vi "ConfigSilos.vi"() -> ()   [LabVIEW 2014]
doc: "The LabJack T7 offers several AIN Extended Features. One such feature is called FlexRMS. Data acquired at a specified AIN Channel are buffered, on-board calculations (rms,range,average) are performed and the results are written to AIN-EF registers. This VI configures the Flex RMS EF to avoid using external computational resources whilst seeking averaged data. THE SCAN DURATION CANNOT EXCEED 180 ms!!"
panel:
  in  "Remote Port":u16=502
  in  "Remote IP Address":string="192.168.126.147"
  in  "Num AI Channels":dbl=16.0
  out "Scan Duration (ms)":dbl=180.0
  in  "Scan Rate (Hz)":sgl=6000.0
  in  "Hysteresis":u32=100
  in  "NumScans":u32=1080
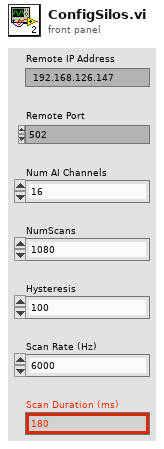
[diagram p1: front panel]
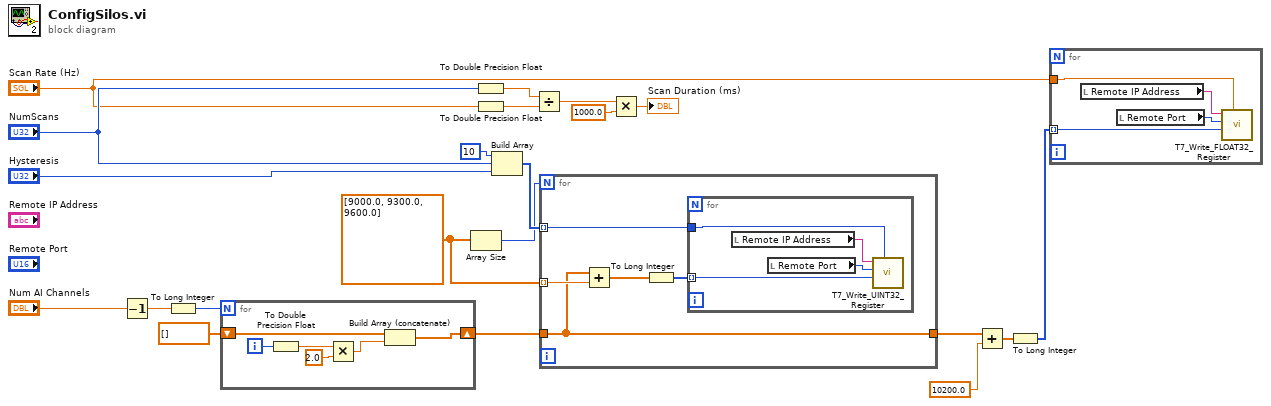
[diagram p0: block diagram]
diagram:
  w13 = dbl[] [9000.0, 9300.0, 9600.0]
  n1 = Decrement(x="Num AI Channels") -> (x-1=w18:dbl)
  n2 = To Long Integer(number=w18) -> (32bit integer=w19:i32)
  n3 = for {
    N: w19 -> [_]
    shift-right: [w26] -> w17
    shift-left: dbl[] [] -> [w25]
    i -> [w27]
    n4 = To Double Precision Float(number=w27) -> (double precision float=w23:dbl)
    n5 = Multiply(x=w23, y=2.0) -> (x*y=w22:dbl)
    n6 = Build Array (concatenate)(w25, w22) -> (w26:dbl[])
  }
  n7 = Array Size(array=w13) -> (size(s)=w12:i32)
  n8 = To Double Precision Float(number="NumScans") -> (double precision float=w3:dbl)
  n9 = To Double Precision Float(number="Scan Rate (Hz)") -> (double precision float=w2:dbl)
  n10 = Build Array(u32 10 ("UINT32 to Write"), "NumScans", "Hysteresis") -> (w14:u32[])
  n11 = Divide(x=w3, y=w2) -> (x/y=w5:dbl)
  n12 = for {
    N: w12 -> [_]
    tunnel: w13 -> [w30] mode=indexing
    tunnel: w17 -> [w28]
    tunnel: w14 -> [w29] mode=indexing
    tunnel: [w28] -> w9
    n13 = Add(x=w28, y=w30) -> (x+y=w31:dbl[])
    n14 = To Long Integer(number=w31) -> (32bit integer=w32:i32[])
    n15 = for {
      tunnel: w32 -> [w35] mode=indexing
      tunnel: w29 -> [w34]
      n16 = local read "Remote IP Address"() -> (w36:string)
      n17 = local read "Remote Port"() -> (w33:u16)
      n18 = call "T7_Write_UINT32_Register.vi"("UINT32 to Write"=w34, "LabJack Test UINT32 Register"=w35, "Remote Port"=w33, "Remote IP Address"=w36) -> ()  [unwired: 8 in]
    }
  }
  n19 = Multiply(x=w5, y=1000.0) -> (x*y=→"Scan Duration (ms)":dbl)
  n20 = Add(x=w9, y=10200.0) -> (x+y=w11:dbl[])
  n21 = To Long Integer(number=w11) -> (32bit integer=w8:i32[])
  n22 = for {
    tunnel: "Scan Rate (Hz)" -> [w39]
    tunnel: w8 -> [w38] mode=indexing
    n23 = local read "Remote IP Address"() -> (w40:string)
    n24 = local read "Remote Port"() -> (w37:u16)
    n25 = call "T7_Write_FLOAT32_Register.vi"("FLOAT32 to Write"=w39, "LabJack TestFLOAT32 Register"=w38, "Remote Port"=w37, "Remote IP Address"=w40) -> ()  [unwired: 8 in]
  }
